vi "Filter DependendentTypeDefs&Parents.vi"(9 "Parent VI Name":string, 10 "Dependency Name":string, 11 "Dependendent TypeDefs wParents":T1[](array[typedef])) -> (2 "Index":i32, 3 "Dependendent TypeDef wParents":T1)   [LabVIEW 2013, in "DiscoverCommonTypeDefCallers.lvlib"]
uses:
  DiscoverCommonTypeDefCallers.lvlib
  DependendentTypeDefswParents.ctl
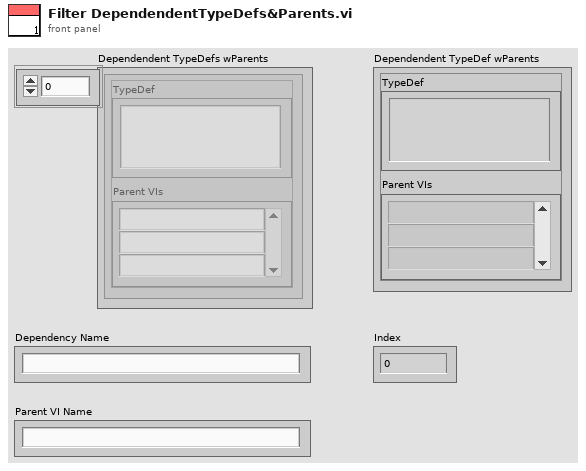
[diagram p1: front panel]
types:
  T1 = typedef "DiscoverCommonTypeDefCallers.lvlib/DependendentTypeDefswParents.ctl" = cluster{"TypeDef":string, "Parent VIs":string[]}
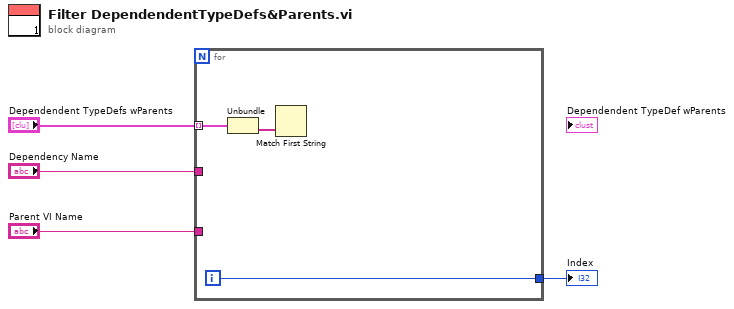
[diagram p0: block diagram]
diagram:
  n1 = for {
    tunnel: "Dependendent TypeDefs wParents" -> [w7] mode=indexing
    tunnel: "Parent VI Name" -> [_]
    tunnel: "Dependency Name" -> [_]
    tunnel: [w5] -> w1
    i -> [w5]
    n2 = Unbundle(w7) -> ("Parent VIs"=w6:string[])  [unwired: 1 out]
    n3 = Match First String(2:w6) -> ()  [unwired: 1 in, 2 out]
  }
  "Index" <- w1
